vi "Determine message source.vi"(11 "message in":string) -> (3 "message out":string, 5 "msg destination":T1)   [LabVIEW 2019, in "Communication Interface.lvlib"]
uses:
  Communication Interface.lvlib
  message destination.ctl
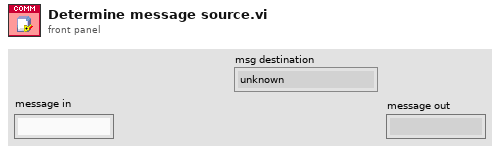
[diagram p1: front panel]
types:
  T1 = typedef "Communication Interface.lvlib/message destination.ctl" = enum16{"unknown", "HW", "Data", "GUI", "Log", "Close"}
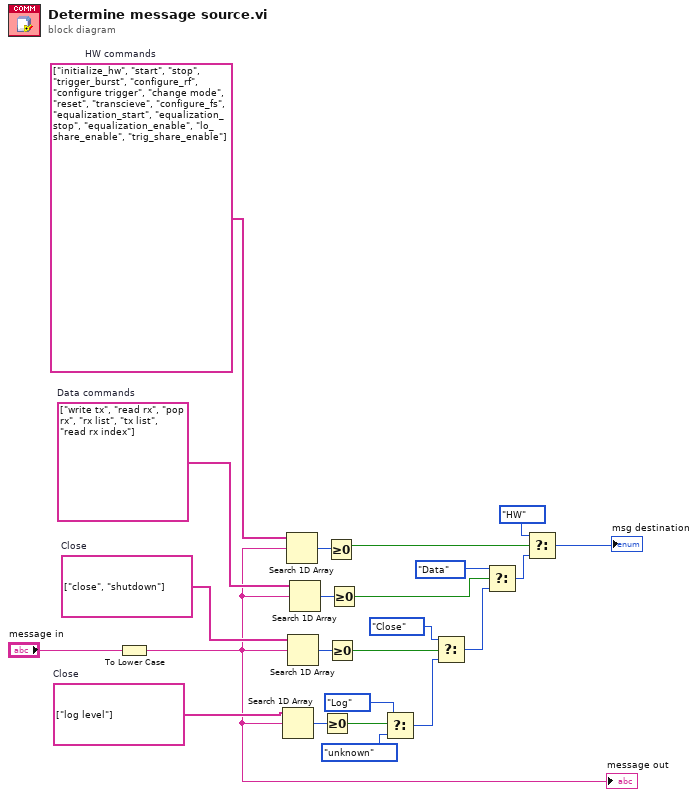
[diagram p0: block diagram]
diagram:
  w6 = string[] ["log level"]  # Close
  w11 = string[] ["close", "shutdown"]  # Close
  w16 = string[] ["write tx", "read rx", "pop rx", "rx list", "tx list", "read rx index"]  # Data commands
  w22 = string[] ["initialize_hw", "start", "stop", "trigger_burst", "configure_rf", "configure trigger", "change mode", "reset", "transcieve", "configure_fs", "equalization_start", "equalization_stop", "equalization_enable", "lo_share_enable", "trig_share_enable"]  # HW commands
  n1 = To Lower Case(string="message in") -> (all lower case string=w5:string)
  "message out" <- w5
  n2 = Search 1D Array(1D array=w6, element=w5) -> (index of element=w7:i32)  [unwired: 1 in]
  n3 = Search 1D Array(1D array=w22, element=w5) -> (index of element=w21:i32)  [unwired: 1 in]
  n4 = Search 1D Array(1D array=w11, element=w5) -> (index of element=w12:i32)  [unwired: 1 in]
  n5 = Search 1D Array(1D array=w16, element=w5) -> (index of element=w17:i32)  [unwired: 1 in]
  n6 = Greater Or Equal To 0?(x=w7) -> (x >= 0?=w3:bool)
  n7 = Greater Or Equal To 0?(x=w21) -> (x >= 0?=w20:bool)
  n8 = Greater Or Equal To 0?(x=w12) -> (x >= 0?=w10:bool)
  n9 = Greater Or Equal To 0?(x=w17) -> (x >= 0?=w14:bool)
  n10 = Select(t=message_destination."Log", s=w3, f=message_destination."unknown" ("msg destination")) -> (s? t:f=w1:T1)
  n11 = Select(t=message_destination."Close" ("msg destination"), s=w10, f=w1) -> (s? t:f=w8:T1)
  n12 = Select(t=message_destination."Data" ("msg destination"), s=w14, f=w8) -> (s? t:f=w15:T1)
  n13 = Select(t=message_destination."HW" ("msg destination"), s=w20, f=w15) -> (s? t:f=→"msg destination":T1)
